vi "SwissSPAD Live_Get Actual Image Size.vi"(8 "error in (no error)":errorcluster) -> (0 "error out":errorcluster, 1 "Y size":i32, 3 "X size":i32)   [LabVIEW 2021]
uses:
  SwissSPAD Live_Settings List.ctl
  SwissSPAD Live_SSx PCB Version.ctl
  Variant/Variant to Data/Variant to Data.lvlib
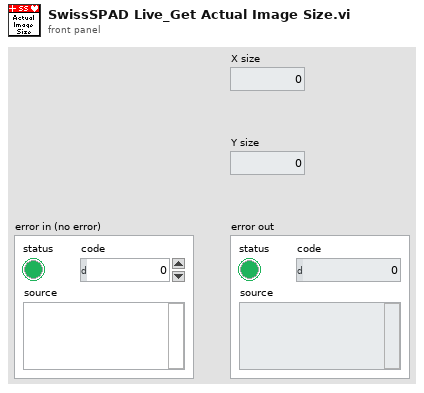
[diagram p1: front panel]
types:
  T1 = typedef "SwissSPAD Live_SSx PCB Version.ctl" = enum16{"unknown", "SS2 PCB1", "SS2 PCB2", "SS3 PCB1"}
  T2 = typedef "SwissSPAD Live_Settings List.ctl" = enum16{"FPGA:Bottom Half", "FPGA:Top Half", "FPGA:Bottom Bitfile Path", "FPGA:Top Bitfile Path", "FPGA:Bottom Bitstream Version", "FPGA:Top Bitstream Version", "FPGA:Auto Reset FPGA", "FPGA:Bottom FPGA Serial Number", "FPGA:Top FPGA Serial Number", "FPGA:Detector PCB Version", "Acquisition Parameters:Microlens", "Acquisition Parameters:SS2 DAQ Parameters", "Acquisition Parameters:Gate Configuration Array", "Acquisition Parameters:SS3 DAQ Parameters", "Acquisition Parameters:Buffer Size (# 8-bit Gates)", "File Information:File Information", "File Information:# Datasets in Series", "File Information:Scrambled File Flag", "File Information:SS3 Gate Slip Correction", "File Information:SS3 Hot Pixel Mismatch Detection", "File Information:Delay between Datasets", "File Information:Save Sum of All Gates Preview", "Image Parameters:Image ROI Information", "Image Parameters:Image Binning Options", "Image Parameters:SS3 Displayed Image", "Image Parameters:Image Display Options", "Image Parameters:Use Histogram Cursors", "Image Parameter:FPGA Data to Display", "UI Settings:Histogram Bins Number", "UI Settings:Histogram Bin Size", "UI Settings:Use Image Display Options", "UI Settings:Verbose Settings", "UI Settings:Verbose Saving"}
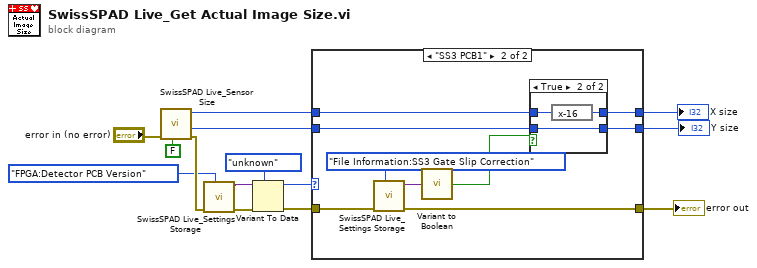
[diagram p0: block diagram]
diagram:
  n1 = call "SwissSPAD Live_Sensor Size.vi"("Set/Get(F)"=FALSE, "Error In"="error in (no error)") -> ("Error Out"=w7:errorcluster, "Y size"=w14:i32, "X size"=w13:i32)  [unwired: 7 in]
  n2 = call "SwissSPAD Live_Settings Storage.vi"("Settings List"=SwissSPAD_Live_Settings_List."FPGA:Detector PCB Version", "Error In"=w7) -> ("Error Out"=w6:errorcluster, "Variant Data out"=w1:variant)  [unwired: 8 in]
  n3 = Variant To Data(error in=w6, type=SwissSPAD_Live_SSx_PCB_Version."unknown" ("Detector PCB Version"), Variant=w1) -> (data=w3:T1, error out=w5:errorcluster)
  n4 = case shown="\"SS3 PCB1\"" w3 {
    tunnel: w14 -> [w16 w26]
    tunnel: w13 -> [w17 w25]
    tunnel: [w15 w23] -> w11
    tunnel: [w16 w22] -> w10
    tunnel: [w17 w21] -> w9
    tunnel: w5 -> [w15 w20]
    frame "unknown", Default {
    }
    frame "SS3 PCB1" {
      n5 = call "SwissSPAD Live_Settings Storage.vi"("Settings List"=SwissSPAD_Live_Settings_List."File Information:SS3 Gate Slip Correction", "Error In"=w20) -> ("Error Out"=w23:errorcluster, "Variant Data out"=w18:variant)  [unwired: 8 in]
      n6 = call "Variant to Boolean.vi"("Variant"=w18) -> ("Value"=w24:bool)  [unwired: 8 in]
      n7 = case shown="True" w24 {
        tunnel: w25 -> [w28 w30]
        tunnel: w26 -> [w27 w31]
        tunnel: [w28 w29] -> w21
        tunnel: [w27 w31] -> w22
        frame False {
        }
        frame True {
          n8 = expression code="x-16"(w30) -> (w29:i32)
        }
      }
    }
  }
  "error out" <- w11
  "Y size" <- w10
  "X size" <- w9
